vi "Create Request.vi"(6 "notification? (F)":bool, 8 "error in (no error)":errorcluster, 9 "params":variant, 10 "method":string) -> (0 "error out":errorcluster, 2 "<JSON> Requests":string, 3 "JSON-RPC out":refnum<class "JSON-RPC.lvclass">, 4 "IDs":string)   [LabVIEW 2019, in "JSON-RPC.lvclass"]
doc: "Format a Request object to send to a Server.\n\n<b>method</b> is a String containing the name of the method to be involked. Method names begining with \"rpc.\" are reserved for rpc-internal methods and extensions.\n\n<b>params</b> is a Structured value. The object will be formatted as follows:\n- Clusters will be flattened to json by-name\n- Arrays will be converted to json array\n- Elements (string, float, etc) will be converted to a 1 element json array\n\n<b>notification?</b> controls whether or not an id will be generated and sent. Requests without an id are treated as a notification and will not be responded to.\n\n<b>Note:</b> While the JSON-RPC spec supports batch Requests, this library currently does not have this feature.\n\nhttps://www.jsonrpc.org/specification"
uses:
  JSON-RPC.lvclass
  typedefs/Request--Cluster.ctl
  JSON-RPC.lvclass/JSON-RPC.ctl
  <vilib>/JDP Science/JSONtext/Make JSON Object.vi
  private/Create ID.vi
  private/Variant to JSON.vi
  <vilib>/Utility/MD5Checksum.llb/MD5Checksum string.vi
  <vilib>/JDP Science/JSONtext/support/Format JSON Object.vi
  <vilib>/JDP Science/JSONtext/support/Format JSON Array Text.vi
  <vilib>/JDP Science/JSONtext/JSONtext.lvlib
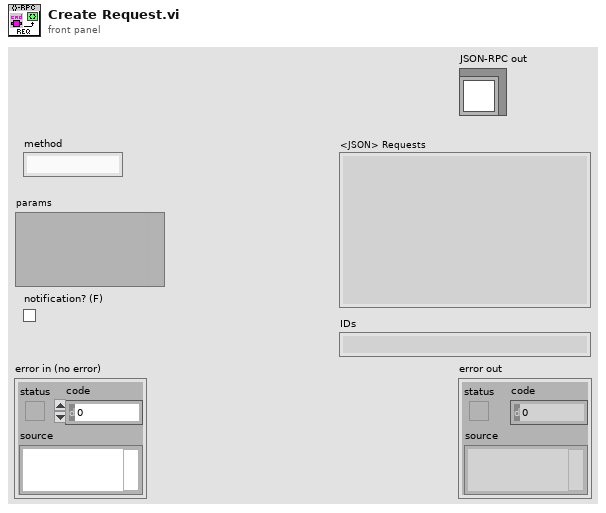
[diagram p1: front panel]
types:
  T1 = typedef "JSON-RPC.lvclass/Request--Cluster.ctl" = cluster{"jsonrpc":string, "method":string, "params":string, "id":string}
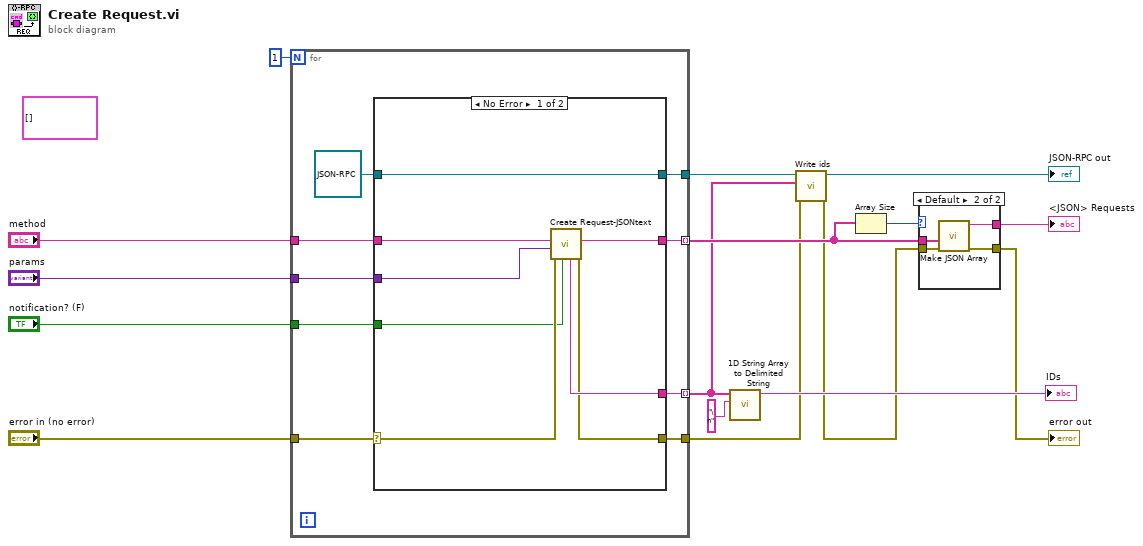
[diagram p0: block diagram]
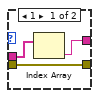
[diagram p3: hidden frame]
diagram:
  (unwired) T1[] [] ("Requests")
  n1 = for {
    N: 1 -> [_]
    tunnel: [w23] -> w7
    tunnel: [w22] -> w12 mode=indexing
    tunnel: [w21] -> w5 mode=indexing
    tunnel: "error in (no error)" -> [w25]
    tunnel: [w24] -> w9
    tunnel: "notification? (F)" -> [w19]
    tunnel: "method" -> [w18]
    tunnel: "params" -> [w17]
    n2 = case shown="No Error" w25 {
      selector: w25 -> [w33 w35]
      tunnel: [w29 w35] -> w24
      tunnel: [w30 w34] -> w23
      tunnel: refnum<class "JSON-RPC.lvclass"> refnum ("JSON-RPC in") -> [w30 w34]
      tunnel: [w31 _] -> w22
      tunnel: [w32 _] -> w21
      tunnel: w19 -> [w28 _]
      tunnel: w18 -> [w27 _]
      tunnel: w17 -> [w26 _]
      frame No Error {
        n3 = call "Create Request-JSONtext.vi"("notification?"=w28, "error in (no error)"=w33, "params"=w26, "method"=w27) -> ("error out"=w29:errorcluster, "<JSON>"=w31:string, "id"=w32:string)  [unwired: 5 in]
      }
      frame Error {
      }
    }
  }
  n4 = call <vilib>:"1D String Array to Delimited String.vi"("delimiter"="\n", "string array"=w5) -> ("delimited string"=→"IDs":string)  [unwired: 9 in]
  n5 = call "Write ids.vi"("error in (no error)"=w9, "ids"=w5, "JSON-RPC in"=w7) -> ("error out"=w8:errorcluster, "JSON-RPC out"=→"JSON-RPC out":refnum<class "JSON-RPC.lvclass">)  [unwired: 7 in]
  n6 = Array Size(array=w12) -> (size(s)=w10:i32)
  n7 = case shown="Default" w10 {
    tunnel: [w37 w42] -> w15
    tunnel: w12 -> [w36 w41]
    tunnel: [w38 w40] -> w11
    tunnel: w8 -> [w38 w39]
    frame 1 {
      n8 = Index Array(array=w36) -> (element=w37:string)  [unwired: 1 in]
    }
    frame Default {
      n9 = call <vilib>:"Make JSON Array.vi"("error in (no error)"=w39, "JSON Elements"=w41) -> ("error out"=w40:errorcluster, "<JSON>"=w42:string)  [unwired: 8 in]
    }
  }
  "error out" <- w11
  "<JSON> Requests" <- w15
